vi "5.-SubVI (Subrutina).vi"() -> ()   [LabVIEW 2020]
panel:
  out "Fecha y hora":string
  in  "Rango de muestreo en milisegundos":dbl
  out "Puntos adquiridos":i32
  in  "Puntos a adquirir":i32
  out "Temperatura":cluster{"señal":dbl, "Limite superior":dbl}(graph)
  out "Fuera de rango":bool
  in  "Limite superior":dbl
  in  "stop":bool
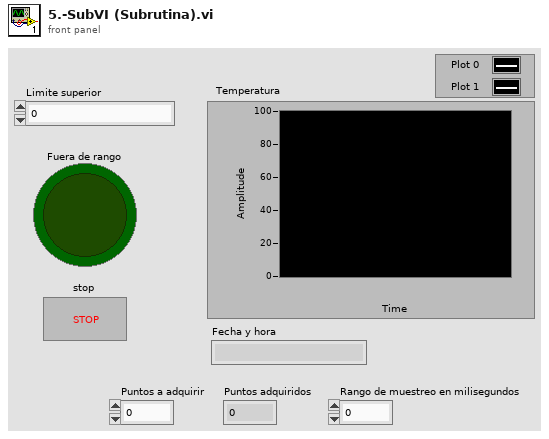
[diagram p1: front panel]
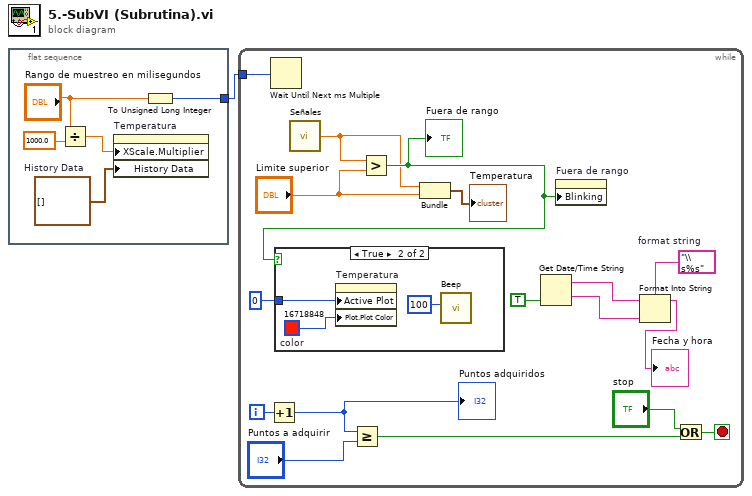
[diagram p0: block diagram]
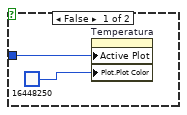
[diagram p2: hidden frame]
diagram:
  n1 = flat-sequence {
    tunnel: [w3] -> w1
    frame #0 {
      w6 = cluster{"señal":dbl, "Limite superior":dbl}[] []  # History Data
      n2 = Divide(x="Rango de muestreo en milisegundos", y=1000.0) -> (x/y=w4:dbl)
      n3 = property on="Temperatura" class="WFChart (strict)"("XScale.Multiplier"=w4, "History Data"=w6) -> ()  [unwired: 2 in, 2 out]
      n4 = To Unsigned Long Integer(number="Rango de muestreo en milisegundos") -> (unsigned 32bit integer=w3:u32)
    }
  }
  n5 = while {
    tunnel: w1 -> [w13]
    i -> [w21]
    stop <- w16 stop-if-true
    w9 = "\\s%s"  # format string
    n6 = Increment(x=w21) -> (x+1=w20:i32)
    "Puntos adquiridos" <- w20
    n7 = Wait Until Next ms Multiple(millisecond multiple=w13) -> ()  [unwired: 1 out]
    n8 = call "Señales.vi"() -> ("Señal"=w7:dbl)
    n9 = Greater Or Equal?(x=w20, y="Puntos a adquirir") -> (x >= y?=w17:bool)
    n10 = Greater?(x=w7, y="Limite superior") -> (0:w15:bool)
    "Fuera de rango" <- w15
    n11 = case shown="True" w15 {
      tunnel: u32 0 -> [w25 w28]
      frame False {
        n12 = property on="Temperatura" class="WFChart (strict)"("Active Plot"=w25, "Plot.Plot Color"=u32 16448250) -> ()  [unwired: 2 in, 2 out]
      }
      frame True {
        w27 = u32 16718848  # color
        n13 = property on="Temperatura" class="WFChart (strict)"("Active Plot"=w28, "Plot.Plot Color"=w27) -> ()  [unwired: 2 in, 2 out]
        n14 = call <vilib>:"Beep.vi"("duration (msec)"=u32 100) -> ()  [unwired: 11 in]
      }
    }
    n15 = Bundle "Bundle"("Señal"=w7, "Limite superior"="Limite superior") -> (→"Temperatura":cluster{"Señal":dbl, "Limite superior":dbl})  [unwired: 1 in]
    n16 = Get Date/Time String(want seconds? (F)=TRUE) -> (date string=w11:string, time string=w10:string)  [unwired: 2 in]
    n17 = property on="Fuera de rango" class="Bool (strict)"("Blinking"=w15) -> ()  [unwired: 2 in, 2 out]
    n18 = Format Into String "Format Into String"(format string=w9, initial string=w11, w10) -> (resulting string=→"Fecha y hora":string)  [unwired: 1 in, 1 out]
    n19 = Or(x="stop", y=w17) -> (x .or. y?=w16:bool)
  }
